vi "Do Request.vi"(7 "Processing In":refnum<class "Processing.lvclass">, 11 "TimerActionController in":refnum<class "TimerActionController.lvclass">) -> (0 "error out":errorcluster, 5 "Processing":refnum<class "Processing.lvclass">)   [LabVIEW 2020, in "Timer Demo.lvlib" / "TimerActionController.lvclass"]
uses:
  TimerActionController.lvclass
  TimerActionController.lvclass/TimerActionController.ctl
  Timer Action Response.ctl
  Timer Demo.lvlib
  lv-stream/stream/URI/URI.lvclass
  lv-http-util/HTTP Utils/Request/Request.lvclass
  lv-http-server/HTTP Server/Processing/Processing.lvclass
  Timer Action.ctl
  Timer Action Request.ctl
  lv-http-util/HTTP Utils/Response/Response.lvclass
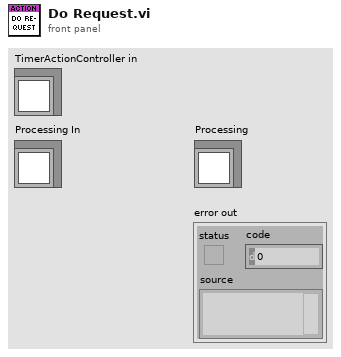
[diagram p1: front panel]
types:
  T1 = typedef "Timer Demo.lvlib/Timer Action.ctl" = enum16{"start", "pause", "reset"}
  T2 = typedef "Timer Demo.lvlib/Timer Action Request.ctl" = cluster{"Timer Action":T1, "Response":refnum<notifier>}
  T3 = typedef "Timer Demo.lvlib/Timer Action Response.ctl" = cluster{"Error":errorcluster}
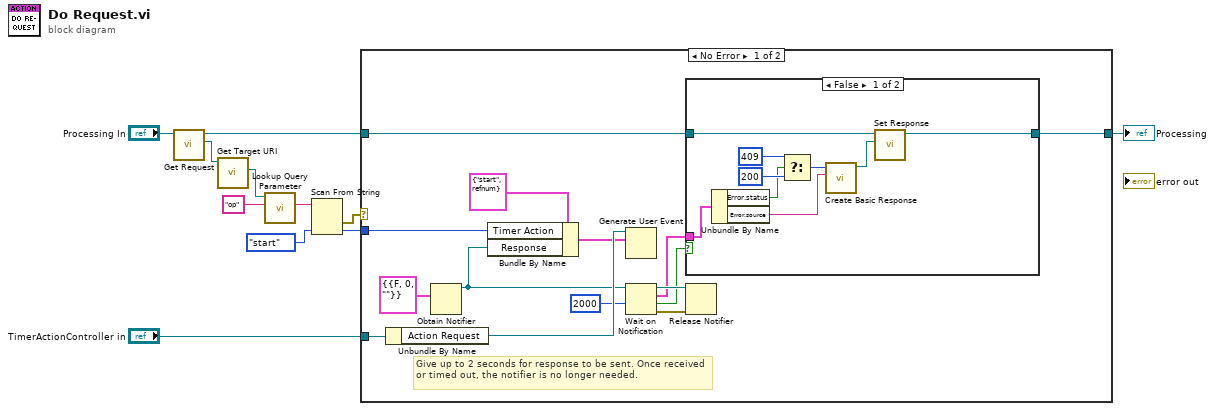
[diagram p0: block diagram]
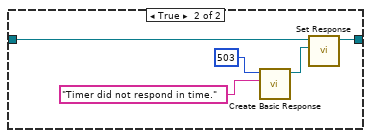
[diagram p2: hidden frame]
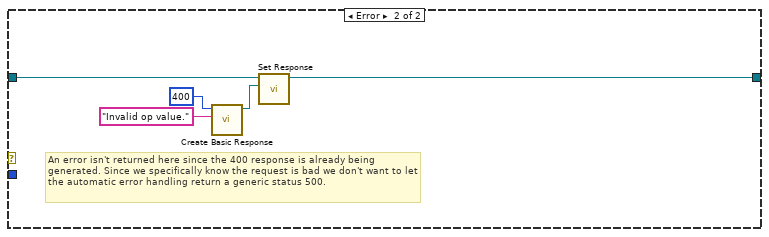
[diagram p3: hidden frame]
diagram:
  n1 = call "Get Request.vi"("Processing in"="Processing In") -> ("Request"=w10:refnum<class "Request.lvclass">, "Processing out"=w3:refnum<class "Processing.lvclass">)  [unwired: 9 in]
  n2 = call "Get Target URI.vi"("Request in"=w10) -> ("Target URI"=w9:refnum<class "URI.lvclass">)  [unwired: 8 in, 2 out]
  n3 = call "Lookup Query Parameter.vi"("Name"="op", "URI in"=w9) -> ("Value"=w7:string)  [unwired: 6 in, 3 out]
  n4 = Scan From String(input string=w7, default 1=Timer_Action."start" ("Timer Action")) -> (error out=w5:errorcluster, output 1=w4:T1)  [unwired: 3 in, 2 out]
  n5 = case shown="No Error" w5 {
    tunnel: w4 -> [w20 _]
    tunnel: w3 -> [w13 w42]
    tunnel: "TimerActionController in" -> [w24 _]
    tunnel: [w12 w40] -> w1
    frame No Error {
      # "Give up to 2 seconds for response to be sent. Once received or timed out, the notifier is no longer needed."
      n6 = Unbundle By Name(w24) -> ("Action Request"=w23:refnum<user-event>)
      n7 = Obtain Notifier(notification data type=T3 {"Error"={"status"=FALSE, "code"=0, "source"=""}} ("Timer Action Response")) -> (notifier out=w19:refnum<notifier>)  [unwired: 3 in, 2 out]
      n8 = Bundle By Name(cluster=T2 {"Timer Action"=enum."start", "Response"=refnum} ("event data"), "Timer Action"=w20, "Response"=w19) -> (w21:T2)
      n9 = Generate User Event(user event=w23, event data cluster=w21) -> ()  [unwired: 2 in, 2 out]
      n10 = Wait on Notification(notifier=w19, timeout in ms (-1)=2000) -> (notifier out=w17:refnum<notifier>, notification=w14:T3, timed out?=w15:bool, error out=w16:errorcluster)  [unwired: 2 in]
      n11 = case shown="False" w15 {
        tunnel: w14 -> [w34 _]
        tunnel: w13 -> [w28 w38]
        tunnel: [w26 w37] -> w12
        frame False {
          n12 = Unbundle By Name(w34) -> ("Error.status"=w30:bool, "Error.source"=w32:string)
          n13 = Select(t=u16 409, s=w30, f=u16 200 ("Status Code")) -> (s? t:f=w29:u16)
          n14 = call "Create Basic Response.vi"("Payload"=w32, "Status Code"=w29) -> ("Response out"=w27:refnum<class "Response.lvclass">)  [unwired: 8 in, 1 out]
          n15 = call "Set Response.vi"("Response"=w27, "Processing in"=w28) -> ("Processing out"=w26:refnum<class "Processing.lvclass">)  [unwired: 9 in]
        }
        frame True {
          n16 = call "Create Basic Response.vi"("Payload"="Timer did not respond in time.", "Status Code"=u16 503) -> ("Response out"=w39:refnum<class "Response.lvclass">)  [unwired: 8 in, 1 out]
          n17 = call "Set Response.vi"("Response"=w39, "Processing in"=w38) -> ("Processing out"=w37:refnum<class "Processing.lvclass">)  [unwired: 9 in]
        }
      }
      n18 = Release Notifier(notifier=w17, error in (no error)=w16) -> ()  [unwired: 1 in, 3 out]
    }
    frame Error {
      # "An error isn't returned here since the 400 response is already being generated. Since we specifically know the request is bad we don't want to let the automatic error handling return a generic status 500."
      n19 = call "Create Basic Response.vi"("Payload"="Invalid op value.", "Status Code"=u16 400) -> ("Response out"=w41:refnum<class "Response.lvclass">)  [unwired: 8 in, 1 out]
      n20 = call "Set Response.vi"("Response"=w41, "Processing in"=w42) -> ("Processing out"=w40:refnum<class "Processing.lvclass">)  [unwired: 9 in]
    }
  }
  "Processing" <- w1
